vi "loops.vi"() -> ()   [LabVIEW 2012]
panel:
  out "number (0 to 1) 2":dbl
  out "number (0 to 1)":dbl
  out "Iteration 2":i32
  out "Iteration 1":i32
  in  "stop":bool
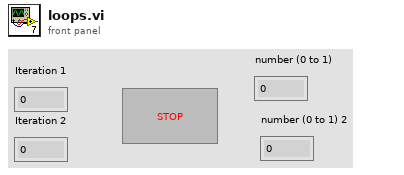
[diagram p1: front panel]
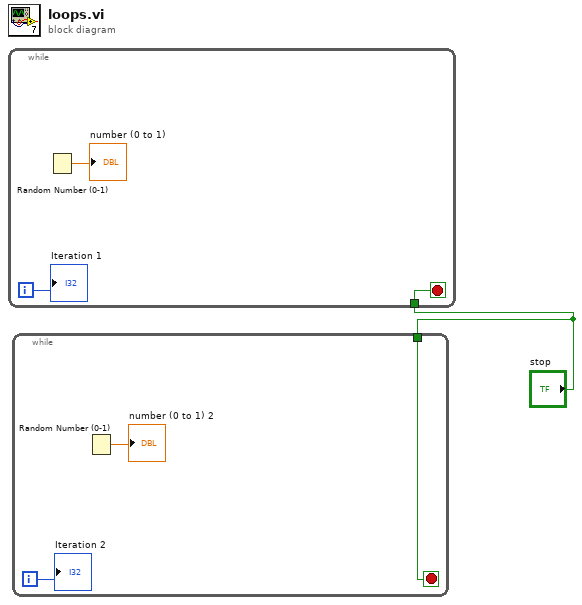
[diagram p0: block diagram]
diagram:
  n1 = while {
    tunnel: "stop" -> [w4]
    i -> [w3]
    stop <- w4 stop-if-true
    n2 = Random Number (0-1)() -> (number: 0 to 1=→"number (0 to 1)":dbl)
    "Iteration 1" <- w3
  }
  n3 = while {
    tunnel: "stop" -> [w7]
    i -> [w6]
    stop <- w7 stop-if-true
    n4 = Random Number (0-1)() -> (number: 0 to 1=→"number (0 to 1) 2":dbl)
    "Iteration 2" <- w6
  }
